vi "Multi-Acq No Objects.vi"(8 "error in":errorcluster, 11 "Synapse CCD in":T1={"JYCCDLib.IJYCCDReqd"=refnum, "JYMONOLib.IJYMonoReqd"=refnum, "Integration time"=0.01, "ADC"=0, "GAIN"=0, "areas :"=[[1, 1, 1, 1024, 256, 1, 256]], "Most Recent Data Object"=refnum, "Mono Properties"={"Grating"=0, "Center Wavelength"=0.0, "Entrance Slit"=0.0, "Exit Slit"=0.0}, "Coverage"={"Max"=0.0, "Min"=0.0}, "Multi-Acquisitions"={"Dark Subtract?"=FALSE, "Averaging?"=FALSE, "Cosmic Ray Removal?"=FALSE, "# to Average"=0, "Time Between Acq."=0, "Acquisitions Control Array"=[TRUE], "Raw Data"=[], "Processed Data"=[], "Array of Wavelengths"=[]}, "Channel Names"=["Wavelength", "Signal"], "Channel Units"=["nm", "counts"]} {"ADC" items=["   20 kHz", "1 MHz", "1 MHz Ultra"]; "GAIN" items=["High Light", "Best Dynamic", "High Sensitivity"]; "Mono Properties"."Grating" items=["1200 lines/mm - 500 nm Blaze", "1200 lines/mm - 750 nm Blaze", "600 lines/mm - 1000 nm Blaze"]}) -> (0 "error out":errorcluster, 3 "Synapse CCD out":T1={"JYCCDLib.IJYCCDReqd"=refnum, "JYMONOLib.IJYMonoReqd"=refnum, "Integration time"=0.01, "ADC"=0, "GAIN"=0, "areas :"=[[1, 1, 1, 1024, 256, 1, 256]], "Most Recent Data Object"=refnum, "Mono Properties"={"Grating"=0, "Center Wavelength"=0.0, "Entrance Slit"=0.0, "Exit Slit"=0.0}, "Coverage"={"Max"=0.0, "Min"=0.0}, "Multi-Acquisitions"={"Dark Subtract?"=FALSE, "Averaging?"=FALSE, "Cosmic Ray Removal?"=FALSE, "# to Average"=0, "Time Between Acq."=0, "Acquisitions Control Array"=[TRUE], "Raw Data"=[], "Processed Data"=[], "Array of Wavelengths"=[]}, "Channel Names"=["Wavelength", "Signal"], "Channel Units"=["nm", "counts"]} {"ADC" items=["   20 kHz", "1 MHz", "1 MHz Ultra"]; "GAIN" items=["High Light", "Best Dynamic", "High Sensitivity"]; "Mono Properties"."Grating" items=["1200 lines/mm - 500 nm Blaze", "1200 lines/mm - 750 nm Blaze", "600 lines/mm - 1000 nm Blaze"]})   [LabVIEW 2009]
doc: "Perform multiple CCD acquisitions in succession.\nUse Setup Multi Acq.vi to properly setup multiple acquisitions."
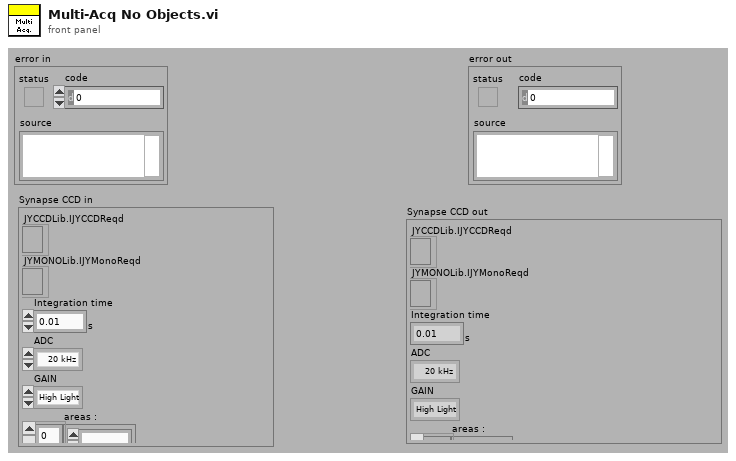
[diagram p1: front panel]
types:
  T1 = cluster{"JYCCDLib.IJYCCDReqd":refnum<k7>, "JYMONOLib.IJYMonoReqd":refnum<k7>, "Integration time":dbl[unit], "ADC":u16, "GAIN":u16, "areas :":i32[][], "Most Recent Data Object":refnum<k7>, "Mono Properties":cluster{"Grating":u16, "Center Wavelength":dbl[unit], "Entrance Slit":dbl[unit], "Exit Slit":dbl[unit]}, "Coverage":cluster{"Max":dbl[unit], "Min":dbl[unit]}, "Multi-Acquisitions":cluster{"Dark Subtract?":bool, "Averaging?":bool, "Cosmic Ray Removal?":bool, "# to Average":u32, "Time Between Acq.":u32, "Acquisitions Control Array":bool[], "Raw Data":i32[][], "Processed Data":dbl[], "Array of Wavelengths":dbl[]}, "Channel Names":string[], "Channel Units":string[]}
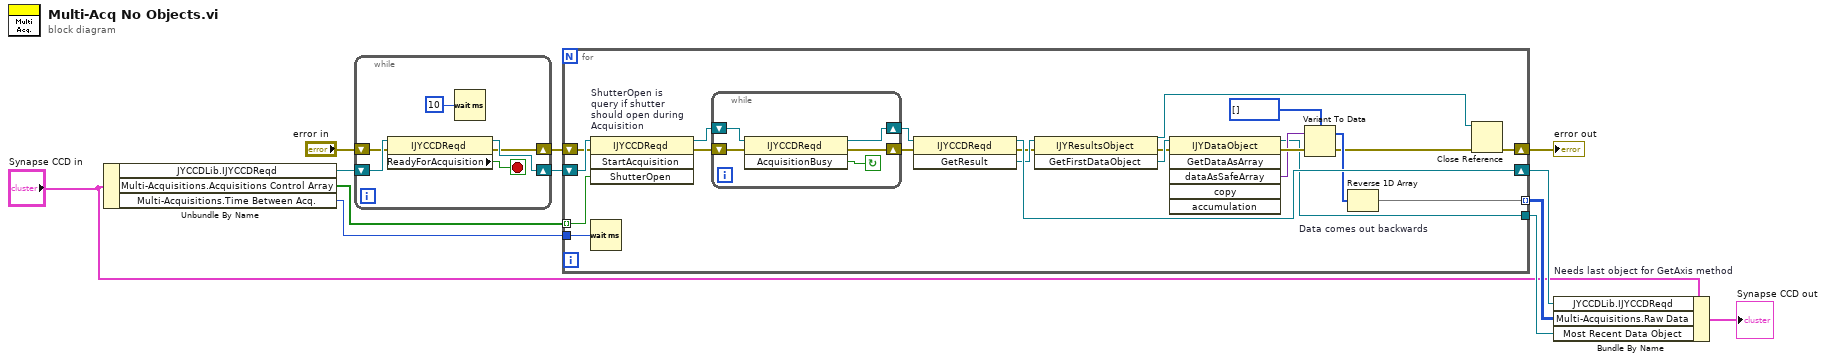
[diagram p0: block diagram]
diagram:
  n1 = Unbundle By Name("Synapse CCD in") -> ("JYCCDLib.IJYCCDReqd"=w5:refnum<k7>, "Multi-Acquisitions.Acquisitions Control Array"=w10:bool[], "Multi-Acquisitions.Time Between Acq."=w9:u32)
  n2 = while {
    shift-right: [w17] -> w4
    shift-left: w5 -> [w18]
    shift-right: [w15] -> w3
    shift-left: "error in" -> [w16]
    stop <- w14 stop-if-true
    n3 = property class="IJYCCDReqd"(reference=w18, error in=w16) -> (reference out=w17:refnum<k7>, error out=w15:errorcluster, "ReadyForAcquisition"=w14:bool)
    n4 = Wait (ms)(milliseconds to wait=u32 10) -> ()  [unwired: 1 out]
  }
  n5 = for {
    shift-right: [w23] -> w12
    shift-left: w3 -> [w35]
    shift-right: [w34] -> w11
    shift-left: w4 -> [w36]
    tunnel: w10 -> [w33] mode=indexing
    tunnel: [w25] -> w8 mode=indexing
    tunnel: w9 -> [w21]
    tunnel: [w19] -> w7
    n6 = invoke on="ShutterOpen is \nquery if shutter\nshould open during\nAcquisition" class="IJYCCDReqd" method="StartAcquisition"(reference=w36, error in=w35, "ShutterOpen"=w33) -> (reference out=w40:refnum<k7>, error out=w39:errorcluster)  [unwired: 1 in, 2 out]
    n7 = Wait (ms)(milliseconds to wait=w21) -> ()  [unwired: 1 out]
    n8 = while {
      shift-right: [w41] -> w38
      shift-left: w39 -> [w42]
      shift-right: [w43] -> w37
      shift-left: w40 -> [w44]
      stop <- w45 continue-if-true
      n9 = invoke class="IJYCCDReqd" method="AcquisitionBusy"(reference=w44, error in=w42) -> (reference out=w43:refnum<k7>, error out=w41:errorcluster, "AcquisitionBusy"=w45:bool)  [unwired: 1 in]
    }
    n10 = invoke class="IJYCCDReqd" method="GetResult"(reference=w37, error in=w38) -> (reference out=w34:refnum<k7>, error out=w31:errorcluster, "GetResult"=w32:refnum<k7>)  [unwired: 1 in]
    n11 = invoke class="IJYResultsObject" method="GetFirstDataObject"(reference=w32, error in=w31) -> (reference out=w22:refnum<k7>, error out=w24:errorcluster, "GetFirstDataObject"=w26:refnum<k7>)  [unwired: 1 in]
    n12 = invoke class="IJYDataObject" method="GetDataAsArray"(reference=w26, error in=w24) -> (reference out=w19:refnum<k7>, error out=w29:errorcluster, "dataAsSafeArray"=w27:variant)  [unwired: 4 in, 3 out]
    n13 = Variant To Data(error in=w29, Variant=w27, type=i32[] []) -> (error out=w20:errorcluster, data=w30:i32[])
    n14 = Reverse 1D Array "Data comes out backwards"(array=w30) -> (reversed array=w25:i32[])
    n15 = Close Reference(reference=w22, error in (no error)=w20) -> (error out=w23:errorcluster)
  }
  "error out" <- w12
  n16 = Bundle By Name "Needs last object for GetAxis method"(cluster="Synapse CCD in", "JYCCDLib.IJYCCDReqd"=w11, "Multi-Acquisitions.Raw Data"=w8, "Most Recent Data Object"=w7) -> (→"Synapse CCD out":T1)
